vi "kleur verkeerslicht.vi"(8 "error in (no error)":errorcluster) -> (0 "error out":errorcluster, 3 "rood licht":bool)   [LabVIEW 2019]
uses:
  <vilib>/myRIO/Instrument Drivers/Onboard IO/I2C/typedefs/I2C Transfer Rate.ctl
  <vilib>/myRIO/Instrument Drivers/Onboard IO/I2C/I2C.lvlib
  <vilib>/myRIO/Instrument Drivers/Onboard IO/I2C/typedefs/I2C User Configuration.ctl
  <vilib>/myRIO/Instrument Drivers/Onboard IO/I2C/typedefs/I2C Configuration.ctl
  <vilib>/myRIO/Common/Instrument Driver Framework/myRIO v1.0/I2C/typedefs/I2C Channels Enum.ctl
  <vilib>/myRIO/Common/Instrument Driver Framework/Utilities/typedefs/Generic FPGA Reference.ctl
  <vilib>/myRIO/Common/Instrument Driver Framework/Utilities/typedefs/myRIO v1.0 Reference.ctl
  <vilib>/myRIO/Common/Instrument Driver Framework/Utilities/typedefs/Hardware Version Enum.ctl
  <vilib>/myRIO/Common/Instrument Driver Framework/Utilities/typedefs/myRIO Generic Hardware Reference.ctl
  <vilib>/myRIO/Instrument Drivers/Onboard IO/I2C/typedefs/I2C Reference.ctl
  <vilib>/myRIO/Instrument Drivers/Onboard IO/I2C/vis/Configure.vi
  <vilib>/myRIO/Instrument Drivers/Onboard IO/I2C/vis/Write.vi
  <vilib>/userDefined/High Color/nirio_resource_hc.ctl
  <vilib>/myRIO/Common/Instrument Driver Framework/myRIO v1.0/I2C/vis/myRIO v1.1 Open I2C.vi
  <vilib>/myRIO/Instrument Drivers/Onboard IO/I2C/vis/myRIO I2C Open.xnode
  <vilib>/myRIO/Common/Instrument Driver Framework/Utilities/vis/Is FPGA Ref Available.vi
  <vilib>/myRIO/Express VI/Onboard IO/I2C/I2C Express VI.xnode
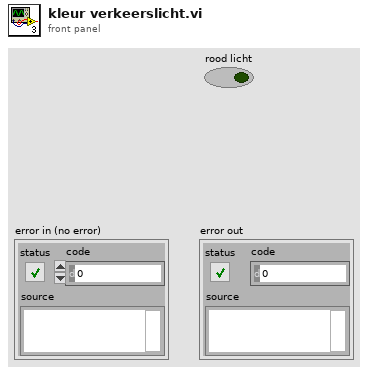
[diagram p1: front panel]
types:
  T1 = typedef "I2C.lvlib/I2C Reference.ctl" = cluster{"myRIO Reference":T2, "I2C Channels Enum":T6, "I2C Configuration":T7}
  T2 = typedef "myRIO Generic Hardware Reference.ctl" = cluster{"myRIO Model":T3, "myRIO Hardware Reference":T4}
  T3 = typedef "Hardware Version Enum.ctl" = enum16{"Unknown", "myRIO-1900", "myRIO-1950", "roboRIO", "NI ELVIS RIO CM", "ELVIS III"}
  T4 = typedef "myRIO v1.0 Reference.ctl" = cluster{"Generic FPGA Reference":T5, "Allow multiple opens":bool}
  T5 = typedef "Generic FPGA Reference.ctl" = refnum<k20>
  T6 = typedef "I2C Channels Enum.ctl" = enum16{"Not Connected", "A/I2C", "B/I2C", "I2C/I2C"}
  T7 = typedef "I2C.lvlib/I2C Configuration.ctl" = cluster{"I2C Transfer Rate":T8}
  T8 = typedef "I2C.lvlib/I2C Transfer Rate.ctl" = enum16{"Standard mode (100 kbps)", "Fast mode (400 kbps)"}
  T9 = typedef "I2C.lvlib/I2C User Configuration.ctl" = cluster{"I2C Transfer Rate":T8}
  T10 = typedef "nirio_resource_hc.ctl" = tag
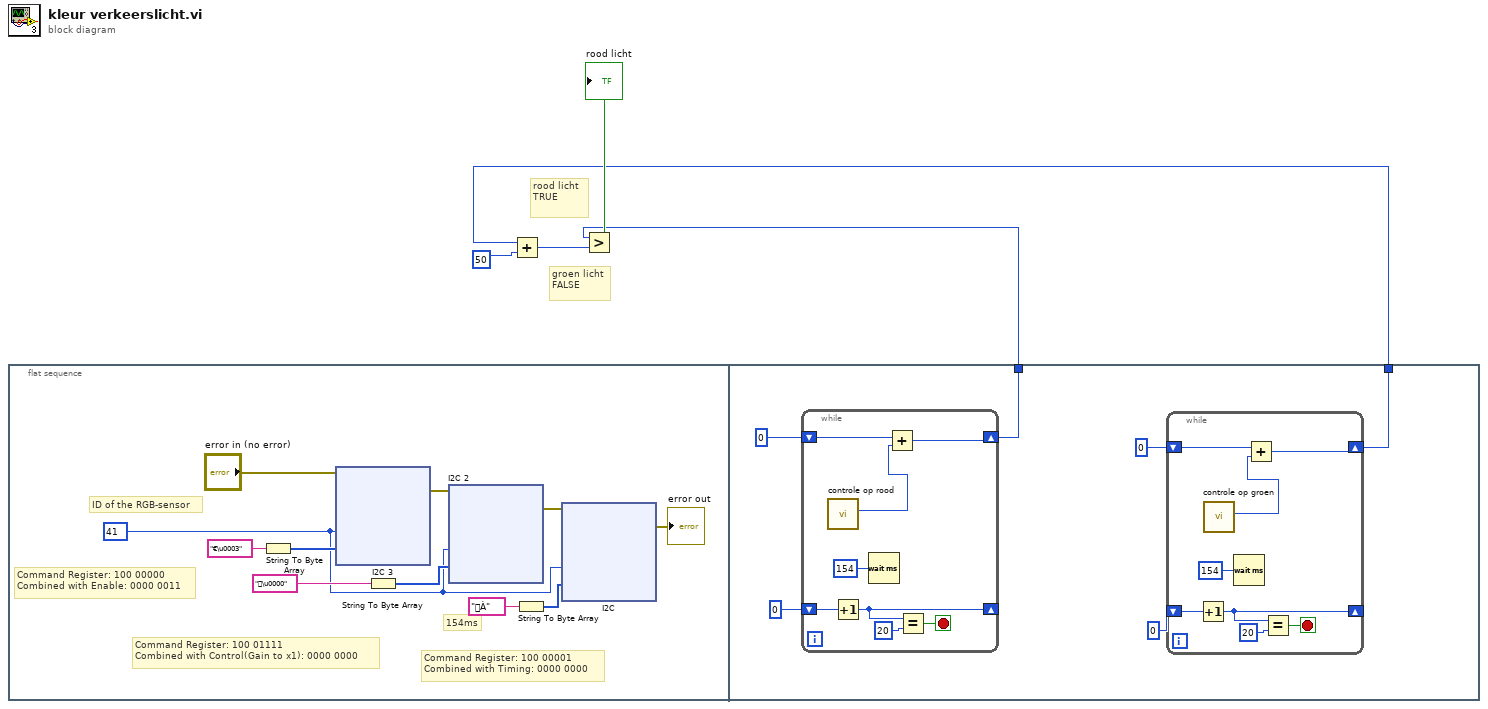
[diagram p0: block diagram]
diagram:
  # "groen licht FALSE"
  # "rood licht TRUE"
  n1 = flat-sequence {
    tunnel: [w132] -> w3
    tunnel: [w131] -> w4
    frame #0 {
      w10 = 41 ("Numeric")
      # "154ms"
      # "ID of the RGB-sensor"
      # "Command Register: 100 00000\nCombined with Enable: 0000 0011"
      # "Command Register: 100 01111\nCombined with Control(Gain to x1): 0000 0000"
      # "Command Register: 100 00001\nCombined with Timing: 0000 0000"
      n2 = String To Byte Array(string="€\u0003") -> (unsigned byte array=w13:u8[])
      n3 = xnode "I2C 3"("Slave Address (7-bit)"=w10, "Bytes to Write"=w13, "error in (no error)"="error in (no error)") -> ("error out"=w9:errorcluster)
      n4 = String To Byte Array(string="\u0000") -> (unsigned byte array=w12:u8[])
      n5 = xnode "I2C 2"("Slave Address (7-bit)"=w10, "Bytes to Write"=w12, "error in (no error)"=w9) -> ("error out"=w8:errorcluster)
      n6 = String To Byte Array(string="À") -> (unsigned byte array=w11:u8[])
      n7 = xnode "I2C"("Slave Address (7-bit)"=w10, "Bytes to Write"=w11, "error in (no error)"=w8) -> ("error out"=→"error out":errorcluster)
    }
    frame #1 {
      n8 = while {
        shift-right: [w149] -> _
        shift-left: 0 -> [w151]
        shift-right: [w145] -> w131
        shift-left: 0 -> [w147]
        stop <- w150 stop-if-true
        n9 = call "controle op rood.vi"() -> ("Total 2"=w146:u32)  [unwired: 8 in, 3 out]
        n10 = Increment(x=w151) -> (x+1=w149:i32)
        n11 = Wait (ms)(milliseconds to wait=u32 154) -> ()  [unwired: 1 out]
        n12 = Add(x=w147, y=w146) -> (x+y=w145:u32)
        n13 = Equal?(x=w149, y=20) -> (x = y?=w150:bool)
      }
      n14 = while {
        shift-right: [w141] -> _
        shift-left: 0 -> [w143]
        shift-right: [w137] -> w132
        shift-left: 0 -> [w138]
        stop <- w142 stop-if-true
        n15 = Increment(x=w143) -> (x+1=w141:i32)
        n16 = call "controle op groen.vi"() -> ("Total"=w139:u32)  [unwired: 8 in, 3 out]
        n17 = Wait (ms)(milliseconds to wait=u32 154) -> ()  [unwired: 1 out]
        n18 = Add(x=w138, y=w139) -> (x+y=w137:u32)
        n19 = Equal?(x=w141, y=20) -> (x = y?=w142:bool)
      }
    }
  }
  n20 = Add(x=w3, y=50) -> (x+y=w1:u32)
  n21 = Greater?(x=w4, y=w1) -> (0:→"rood licht":bool)
